vi "Vision Processing.vi"(4 "error in (no error)":errorcluster, 7 "Image Size":T1=enum."160x120") -> ()   [LabVIEW 2016]
doc: "This VI runs in parallel to other tasks. It gets images from the camera, processes them for color or shape and use that information to affect robot behavior."
uses:
  Program Files (x86)/National Instruments/LabVIEW 2016/examples/FRC/roboRIO/Vision/2017 Vision Example/Vision Support Code/Camera Types.ctl
  <vilib>/Rock Robotics/WPI/Camera/WPI_CameraImageSize.ctl
  <vilib>/Rock Robotics/WPI/Camera/WPI_CameraWhite Balance Values.ctl
  <vilib>/Rock Robotics/WPI/Camera/WPI_CameraExposure Values.ctl
  <vilib>/Rock Robotics/WPI/Camera/WPI_CameraFrameRate.ctl
  Robot Global Data.vi
  <vilib>/vision/NI_Vision_Development_Module.lvlib
panel:
  in  "Image Size 3":T1=enum."160x120"
  in  "LED Color":T2={"Hue"={121.0, 119.0}, "Sat"={176.07142857142858, 255.0}, "Val"={40.53571428571429, 255.0}} {"Hue" scale=0.0..255.0 scale format="%#_3g"}
  out "Qualified Particles":i32
  out "Results":T3 {"Score" format="%#_3g"; "Pixels"."Rectangle"."Numeric 5" format="%#_3g"; "Pixels"."Rectangle"."Numeric 3" format="%#_3g"; "Pixels"."Rectangle"."Numeric 2" format="%#_3g"; "Pixels"."Rectangle"."Numeric" format="%#_3g"; "Normalized"."Rectangle"."Numeric 5" format="%#_2g"; "Normalized"."Rectangle"."Numeric 3" format="%#_2g"; "Normalized"."Rectangle"."Numeric 2" format="%#_2g"; "Normalized"."Rectangle"."Numeric" format="%#_2g"; "Normalized"."Center"."?" format="%#_3g"; "Normalized"."Center"."?" format="%#_3g"; "Distance (ft)" format="%#_3g"}
  in  "Camera Type":T4=enum."MS HD3000 square"
  in  "Score Cutoff %":dbl=70.0
  in  "Particles":dbl=5.0
  in  "Color Mode":u16(ring)=3 items=["RGB", "HSL", "HSV", "HSI"]
  in  "Use Calibration":bool=TRUE
  out "Calibration error":errorcluster
  in  "Line Border":cluster{"Top":dbl, "Bottom":dbl}={"Top"=6.0, "Bottom"=1.0}
  in  "Display Original":bool
  in  "Display Mask":bool
  out "Mask":T5(plugin-control)
  out "Original Image":T5(plugin-control)
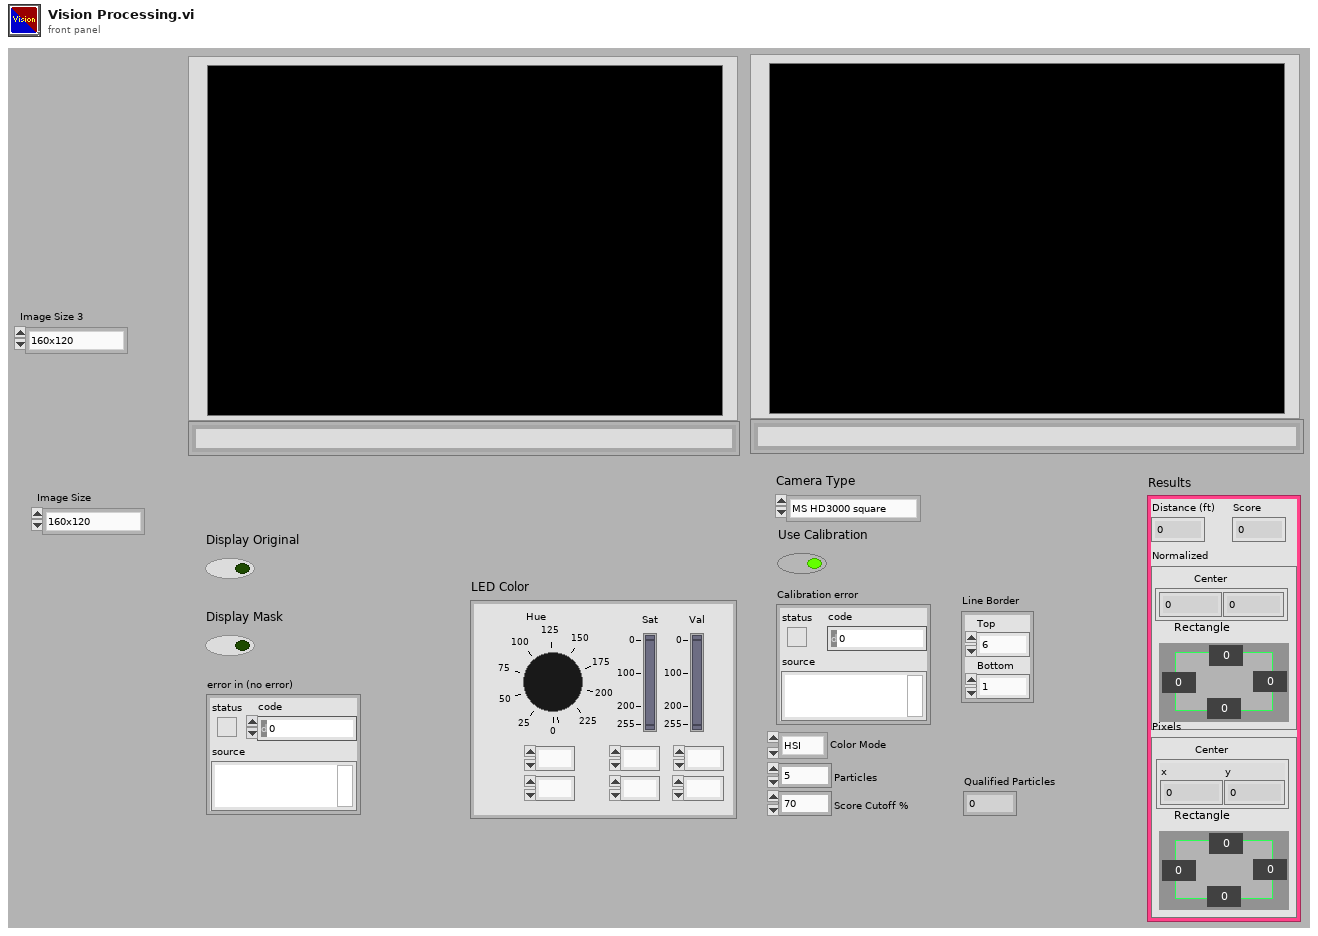
[diagram p1: front panel]
types:
  T1 = typedef "WPI_CameraImageSize.ctl" = enum16{"640x480", "320x240", "160x120", "Custom"}
  T2 = cluster{"Hue":cluster{dbl, dbl}, "Sat":cluster{dbl, dbl}, "Val":cluster{dbl, dbl}}
  T3 = cluster{"Distance (ft)":dbl, "Score":dbl, "Normalized":cluster{"Center":cluster{dbl, dbl}, "Rectangle":cluster{"Numeric":dbl, "Numeric 2":dbl, "Numeric 3":dbl, "Numeric 5":dbl}}, "Pixels":cluster{"Center":cluster{"x":dbl, "y":dbl}, "Rectangle":cluster{"Numeric":dbl, "Numeric 2":dbl, "Numeric 3":dbl, "Numeric 5":dbl}}}
  T4 = typedef "Camera Types.ctl" = enum16{"206", "1011", "1013", "MS HD3000 square", "MS HD3000 640x480"}
  T5 = typedef "IMAQ Image.ctl" = refnum<image>
  T6 = typedef "WPI_CameraFrameRate.ctl" = u32
  T7 = typedef "WPI_CameraExposure Values.ctl" = enum16{"Auto", "Flicker-free 50 Hz", "Flicker-free 60 Hz", "Hold current", "Custom"}
  T8 = typedef "WPI_CameraWhite Balance Values.ctl" = enum16{"Auto", "Fixed indoor", "Fixed outdoor 1", "Fixed outdoor 2", "Fixed fluorescent 1", "Fixed fluorescent 2", "Hold current", "Custom"}
  T9 = typedef "Image Type" = u32
  T10 = typedef "Particle Parameters" = i32
  T11 = typedef "WPI_CameraDevRef.ctl" = cluster{"Camera Address":string, "CameraStatus":errorcluster}
  T12 = cluster{"Left":dbl, "Top":dbl, "Right":dbl, "Bottom":dbl}
  T13 = cluster{"Distance (ft)":dbl, "Score":dbl, "Normalized":cluster{"Center":cluster{dbl, dbl}, "Rectangle":cluster{"Numeric":dbl, "Numeric 2":dbl, "Numeric 3":dbl, "Numeric 5":dbl}}, "Pixels":cluster{"Center":cluster{dbl, dbl}, "Rectangle":cluster{"Numeric":dbl, "Numeric 2":dbl, "Numeric 3":dbl, "Numeric 5":dbl}}}
  T14 = cluster{"Center":cluster{dbl, dbl}, "Rectangle":cluster{"Numeric":dbl, "Numeric 2":dbl, "Numeric 3":dbl, "Numeric 5":dbl}}
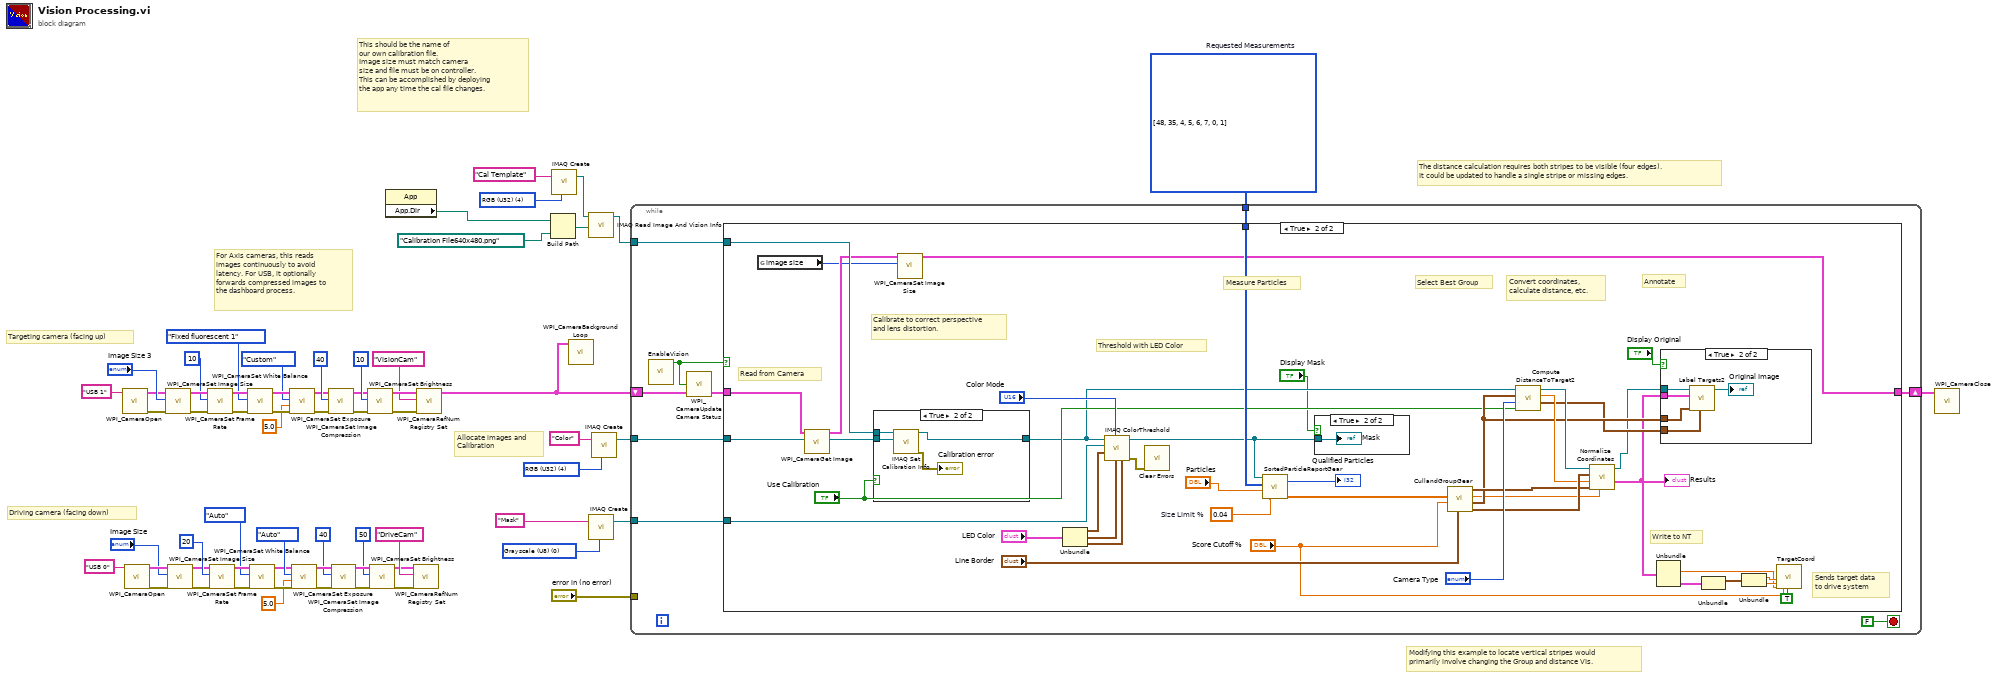
[diagram p0: block diagram]
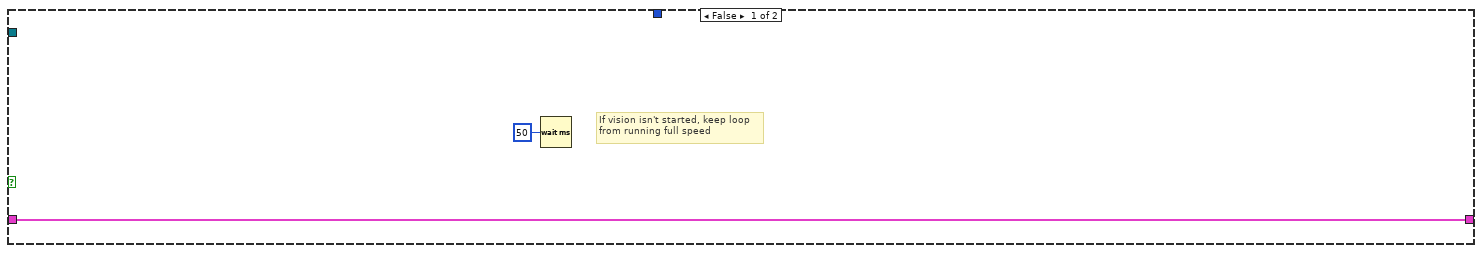
[diagram p2: hidden frame]
diagram:
  w53 = T9 4 items=["Grayscale (U8)", "Grayscale (I16)", "Grayscale (SGL)", "Complex (CSG)", "RGB (U32)", "HSL (U32)", "RGB (U64)", "Grayscale (U16)"] ("Image Type")
  w55 = T9 0 items=["Grayscale (U8)", "Grayscale (I16)", "Grayscale (SGL)", "Complex (CSG)", "RGB (U32)", "HSL (U32)", "RGB (U64)", "Grayscale (U16)"] ("Image Type")
  w56 = T9 4 items=["Grayscale (U8)", "Grayscale (I16)", "Grayscale (SGL)", "Complex (CSG)", "RGB (U32)", "HSL (U32)", "RGB (U64)", "Grayscale (U16)"] ("Image Type")
  w62 = T10[] [48, 35, 4, 5, 6, 7, 0, 1] items=["Center of Mass X", "Center of Mass Y", "First Pixel X", "First Pixel Y", "Bounding Rect Left", "Bounding Rect Top", "Bounding Rect Right", "Bounding Rect Bottom", "Max Feret Diameter Start X", "Max Feret Diameter Start Y", "Max Feret Diameter End X", "Max Feret Diameter End Y", "Max Horiz. Segment Length Left", "Max Horiz. Segment Length Right", "Max Horiz. Segment Length Row", "-", "Bounding Rect Width", "Bounding Rect Height", "Bounding Rect Diagonal", "Perimeter", "Convex Hull Perimeter", "Holes' Perimeter", "Max Feret Diameter", "Equivalent Ellipse Major Axis", "Equivalent Ellipse Minor Axis", "Equivalent Ellipse Minor Axis (Feret)", "Equivalent Rect Long Side", "Equivalent Rect Short Side", "Equivalent Rect Diagonal", "Equivalent Rect Short Side (Feret)", "Average Horiz. Segment Length", "Average Vert. Segment Length", "Hydraulic Radius", "Waddel Disk Diameter", "-", "Area", "Holes' Area", "Particle & Holes' Area", "Convex Hull Area", "Image Area", "-", "Number of Holes", "Number of Horiz. Segments", "Number of Vert. Segments", "-", "Orientation", "Max Feret Diameter Orientation", "-", "% Area/Image Area", "% Area/(Particle & Holes' Area)", "Ratio of Equivalent Ellipse Axes", "Ratio of Equivalent Rect Sides", "-", "Elongation Factor", "Compactness Factor", "Heywood Circularity Factor", "Type Factor", "-", "Sum X", "Sum Y", "Sum XX", "Sum XY", "Sum YY", "Sum XXX", "Sum XXY", "Sum XYY", "Sum YYY", "-", "Moment of Inertia XX", "Moment of Inertia XY", "Moment of Inertia YY", "Moment of Inertia XXX", "Moment of Inertia XXY", "Moment of Inertia XYY", "Moment of Inertia YYY", "Norm. Moment of Inertia XX", "Norm. Moment of Inertia XY", "Norm. Moment of Inertia YY", "Norm. Moment of Inertia XXX", "Norm. Moment of Inertia XXY", "Norm. Moment of Inertia XYY", "Norm. Moment of Inertia YYY", "Hu Moment 1", "Hu Moment 2", "Hu Moment 3", "Hu Moment 4", "Hu Moment 5", "Hu Moment 6", "Hu Moment 7"]  # Requested Measurements
  # "Driving camera (facing down)"
  # "Targeting camera (facing up)"
  # "For Axis cameras, this reads\nimages continuously to avoid\nlatency. For USB, it optionally\nforwards compressed images to\nthe dashboard process."
  # "Allocate images and\nCalibration"
  # "This should be the name of \nour own calibration file.\nImage size must match camera\nsize and file must be on controller.\nThis can be accomplished by deploying\nthe app any time the cal file changes."
  # "Modifying this example to locate vertical stripes would\nprimarily involve changing the Group and distance VIs."
  # "The distance calculation requires both stripes to be visible (four edges).\nIt could be updated to handle a single stripe or missing edges."
  n1 = call <vilib>:"WPI_CameraOpen.vi"("Camera Address"="USB 1" ("format string")) -> ("error out"=w36:errorcluster, "CameraDevRef"=w37:T11)  [unwired: 1 in, 8 out]
  n2 = call <vilib>:"WPI_CameraOpen.vi"("Camera Address"="USB 0" ("format string")) -> ("error out"=w16:errorcluster, "CameraDevRef"=w15:T11)  [unwired: 1 in, 8 out]
  n3 = call <vilib>:"WPI_CameraSet Image Size.vi"("error in (no error)"=w36, "Image Size"="Image Size 3", "CameraDevRef"=w37) -> ("error out"=w35:errorcluster, "CameraDevRef Out"=w38:T11)  [unwired: 1 in, 6 out]
  n4 = call <vilib>:"WPI_CameraSet Image Size.vi"("error in (no error)"=w16, "Image Size"="Image Size", "CameraDevRef"=w15) -> ("error out"=w17:errorcluster, "CameraDevRef Out"=w14:T11)  [unwired: 1 in, 6 out]
  n5 = call <vilib>:"WPI_CameraSet Frame Rate.vi"("error in (no error)"=w35, "Frame Rate (fps)"=T6 10, "CameraDevRef"=w38) -> ("error out"=w34:errorcluster, "CameraDevRef Out"=w40:T11)  [unwired: 7 out]
  n6 = call <vilib>:"WPI_CameraSet Frame Rate.vi"("error in (no error)"=w17, "Frame Rate (fps)"=T6 20, "CameraDevRef"=w14) -> ("error out"=w18:errorcluster, "CameraDevRef Out"=w12:T11)  [unwired: 7 out]
  n7 = call <vilib>:"WPI_CameraSet White Balance.vi"("error in (no error)"=w34, "White Balance"=WPI_CameraWhite_Balance_Values."Fixed fluorescent 1", "CameraDevRef"=w40) -> ("error out"=w33:errorcluster, "CameraDevRef Out"=w39:T11)  [unwired: 1 in, 6 out]
  n8 = call <vilib>:"WPI_CameraSet White Balance.vi"("error in (no error)"=w18, "White Balance"=WPI_CameraWhite_Balance_Values."Auto", "CameraDevRef"=w12) -> ("error out"=w19:errorcluster, "CameraDevRef Out"=w13:T11)  [unwired: 1 in, 6 out]
  n9 = call <vilib>:"WPI_CameraSet Exposure.vi"("error in (no error)"=w33, "Exposure (%)"=5.0 ("f"), "Exposure"=WPI_CameraExposure_Values."Custom", "CameraDevRef"=w39) -> ("error out"=w32:errorcluster, "CameraDevRef Out"=w42:T11)  [unwired: 6 out]
  n10 = call <vilib>:"WPI_CameraSet Exposure.vi"("error in (no error)"=w19, "Exposure (%)"=5.0, "Exposure"=WPI_CameraExposure_Values."Auto", "CameraDevRef"=w13) -> ("error out"=w20:errorcluster, "CameraDevRef Out"=w10:T11)  [unwired: 6 out]
  n11 = call <vilib>:"WPI_CameraSet Image Compression.vi"("error in (no error)"=w32, "Compression"=40, "CameraDevRef"=w42) -> ("error out"=w31:errorcluster, "CameraDevRef Out"=w41:T11)  [unwired: 7 out]
  n12 = call <vilib>:"WPI_CameraSet Image Compression.vi"("error in (no error)"=w20, "Compression"=40, "CameraDevRef"=w10) -> ("error out"=w21:errorcluster, "CameraDevRef Out"=w11:T11)  [unwired: 7 out]
  n13 = call <vilib>:"WPI_CameraSet Brightness.vi"("error in (no error)"=w31, "Brightness"=10, "CameraDevRef"=w41) -> ("error out"=w30:errorcluster, "CameraDevRef Out"=w47:T11)  [unwired: 7 out]
  n14 = call <vilib>:"WPI_CameraSet Brightness.vi"("error in (no error)"=w21, "Brightness"=50, "CameraDevRef"=w11) -> ("error out"=w22:errorcluster, "CameraDevRef Out"=w5:T11)  [unwired: 7 out]
  n15 = property class="App"() -> ("App.Dir"=w48:path)  [unwired: 2 in, 2 out]
  n16 = call <vilib>:"WPI_CameraRefNum Registry Set.vi"("error in (no error)"=w22, "refnum name"="DriveCam", "CameraDevRef"=w5) -> ()  [unwired: 1 in, 8 out]
  n17 = call <vilib>:"WPI_CameraRefNum Registry Set.vi"("error in (no error)"=w30, "refnum name"="VisionCam", "CameraDevRef"=w47) -> ("CameraDevRef"=w1:T11)  [unwired: 1 in, 7 out]
  n18 = Build Path(base path=w48, name or relative path=path "Calibration File640x480.png" ("Folder Location")) -> (appended path=w50:path)
  n19 = call "IMAQ Create"("Image Name"="Cal Template", "Image Type"=w53) -> ("New Image"=w51:T5)  [unwired: 2 in, 2 out]
  n20 = call <vilib>:"WPI_CameraBackground Loop.vi"("CameraDevRef"=w1) -> ()  [unwired: 11 in]
  n21 = call "IMAQ Read Image And Vision Info"("File Path"=w50, "Image"=w51) -> ("Image Out"=w60:T5)  [unwired: 7 in, 2 out]
  n22 = call "IMAQ Create"("Image Name"="Mask", "Image Type"=w55) -> ("New Image"=w63:T5)  [unwired: 2 in, 2 out]
  n23 = call "IMAQ Create"("Image Name"="Color", "Image Type"=w56) -> ("New Image"=w61:T5)  [unwired: 2 in, 2 out]
  n24 = while {
    tunnel: w63 -> [w71]
    tunnel: w62 -> [w70]
    tunnel: w60 -> [w69]
    shift-right: [w68] -> w59
    shift-left: w1 -> [w67]
    tunnel: "error in (no error)" -> [_]
    tunnel: w61 -> [w65]
    stop <- FALSE stop-if-true
    n25 = call "EnableVision.vi"() -> ("EnableVisionOut"=w64:bool)  [unwired: 10 in, 1 out]
    n26 = call <vilib>:"WPI_CameraUpdate Camera Status.vi"("CameraDevRef In"=w67, "Enable Vision"=w64) -> ("CameraDevRef Out"=w66:T11)  [unwired: 3 in]
    n27 = case shown="True" w64 {
      tunnel: w71 -> [_ w116]
      tunnel: w70 -> [_ w112]
      tunnel: w69 -> [_ w98]
      tunnel: [w73 w93] -> w68
      tunnel: w66 -> [w73 w76]
      tunnel: w65 -> [_ w75]
      frame False {
        # "If vision isn't started, keep loop\nfrom running full speed"
        n28 = Wait (ms)(milliseconds to wait=u32 50) -> ()  [unwired: 1 out]
      }
      frame True {
        w111 = 0.04  # Size Limit %
        # "Sends target data\nto drive system"
        # "Write to NT"
        # "Read from Camera"
        # "Calibrate to correct perspective\nand lens distortion."
        # "Measure Particles"
        # "Convert coordinates,\ncalculate distance, etc."
        # "Annotate"
        # "Select Best Group"
        # "Threshold with LED Color"
        n29 = global read "Robot Global Data.vi" "image size"() -> (w77:T1)
        n30 = call <vilib>:"WPI_CameraGet Image.vi"("Image"=w75, "CameraDevRef"=w76) -> ("Image Out"=w95:T5, "CameraDevRef Out"=w94:T11)  [unwired: 7 in, 1 out]
        n31 = case shown="True" "Use Calibration" {
          tunnel: [w123 w127] -> w83
          tunnel: w95 -> [w123 w126]
          tunnel: w98 -> [_ w125]
          frame False {
          }
          frame True {
            n32 = call "IMAQ Set Calibration Info"("Image Dst"=w126, "Image Src"=w125) -> ("error out"=→"Calibration error":errorcluster, "Calibrated Image"=w127:T5)  [unwired: 8 in]
          }
        }
        n33 = call <vilib>:"WPI_CameraSet Image Size.vi"("Image Size"=w77, "CameraDevRef"=w94) -> ("CameraDevRef Out"=w93:T11)  [unwired: 2 in, 7 out]
        n34 = Unbundle("LED Color") -> ("Hue"=w115:cluster{dbl, dbl}, "Sat"=w114:cluster{dbl, dbl}, "Val"=w113:cluster{dbl, dbl})
        n35 = call "IMAQ ColorThreshold"("Blue or Luma or Val or Inten Range"=w113, "Green or Sat Range"=w114, "Color Mode"="Color Mode", "Red or Hue Range"=w115, "Image Dst"=w116, "Image Src"=w83) -> ("error out"=w110:errorcluster, "Image Dst Out"=w107:T5)  [unwired: 4 in]
        n36 = call <vilib>:"Clear Errors.vi"("error in (no error)"=w110) -> ()  [unwired: 5 in, 2 out]
        n37 = call "SortedParticleReportGear.vi"("Min Area Size %"=w111, "Particle Count Limit"="Particles", "Pixel Measurements"=w112, "Image in"=w107) -> ("Sorted Data"=w108:dbl[][], "Particles"=→"Qualified Particles":i32)
        n38 = case shown="True" "Display Mask" {
          tunnel: w107 -> [_ w122]
          frame False {
          }
          frame True {
            "Mask" <- w122
          }
        }
        n39 = call "CullandGroupGear.vi"("Line Border"="Line Border", "Score Cutoff"="Score Cutoff %", "Sorted Data"=w108) -> ("Rect"=w105:T12, "Line"=w99:T12, "Score"=w86:dbl, "Center"=w102:cluster{"X":dbl, "Y":dbl})  [unwired: 5 in]
        n40 = call "Compute DistanceToTarget2.vi"("Calibrated"="Use Calibration", "Camera Type"="Camera Type", "Line"=w99, "Image Src"=w83) -> ("Edges"=w81:cluster{"X":sgl, "Y":sgl}[], "Distance (ft)"=w104:dbl, "Image Dst Out"=w103:T5)  [unwired: 5 in]
        n41 = call "Normalize Coordinates.vi"("Score"=w86, "Center"=w102, "Distance"=w104, "Bounding box"=w105, "Image in"=w103) -> ("Results"=w79:T13, "Image out"=w78:T5)  [unwired: 5 in]
        "Results" <- w79
        n42 = Unbundle(w79) -> ("Score"=w85:dbl, "Pixels"=w92:T14)  [unwired: 2 out]
        n43 = case shown="True" "Display Original" {
          tunnel: w78 -> [_ w121]
          tunnel: w79 -> [_ w120]
          tunnel: w99 -> [_ w119]
          tunnel: w81 -> [_ w118]
          frame False {
          }
          frame True {
            n44 = call "Label Targets2.vi"("Edges"=w118, "Line"=w119, "Results"=w120, "Image in"=w121) -> ("Image out"=→"Original Image":T5)  [unwired: 7 in]
          }
        }
        n45 = Unbundle(w92) -> ("Center"=w91:cluster{dbl, dbl})  [unwired: 1 out]
        n46 = Unbundle(w91) -> (w90:dbl, w89:dbl)
        n47 = call "TargetCoord.vi"("CenterXIn"=w90, "CenterYIn"=w89, "ScoreIn"=w85, "MinScore"="Score Cutoff %", "Update?"=TRUE) -> ()  [unwired: 12 in, 3 out]
      }
    }
  }
  n48 = call <vilib>:"WPI_CameraClose.vi"("CameraDevRef"=w59) -> ()  [unwired: 1 in, 10 out]
